vi "AnalogGetEnabled.vi"(0 "error in (no error)":errorcluster, 2 "index":i32, 3 "Device In":i32) -> (7 "error out":errorcluster, 8 "Enabled?":bool, 9 "EnabledState":i32, 10 "Device Out":i32)   [LabVIEW 2013]
uses:
  phidget21.dll
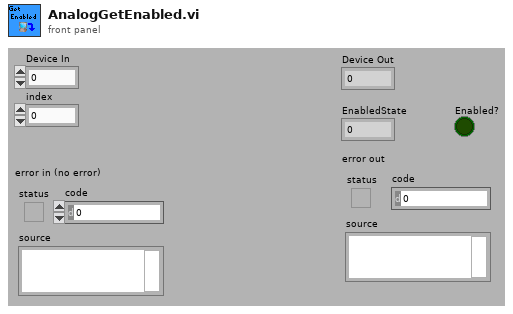
[diagram p1: front panel]
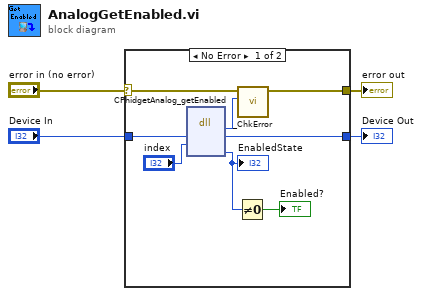
[diagram p0: block diagram]
diagram:
  n1 = case shown="No Error" "error in (no error)" {
    selector: "error in (no error)" -> [w8 w14]
    tunnel: [w7 w14] -> w3
    tunnel: "Device In" -> [w11 w13]
    tunnel: [w10 w13] -> w1
    frame No Error {
      n2 = dll-call lib="phidget21.*" fn="CPhidgetAnalog_getEnabled"("phid"=w11, "index"="index") -> (w9:i32, "phid"=w10:i32, "EnabledState"=w6:i32)  [unwired: 5 in, 2 out]
      "EnabledState" <- w6
      n3 = Not Equal To 0?(x=w6) -> (x != 0?=→"Enabled?":bool)
      n4 = call "_ChkError.vi"("Return Code"=w9, "error in (no error)"=w8) -> ("error out"=w7:errorcluster)  [unwired: 9 in]
    }
    frame Error {
    }
  }
  "error out" <- w3
  "Device Out" <- w1
